vi "Tacking Helper Helper - Starting Angle Test.vi"(6 "Waypoint Array In":T1[](array[typedef]) {"Point Type" items=["Drive", "Round Port", "Round Starboard", "Stay"]}, 9 "Starting Arm Length":dbl, 10 "Tests whether the while\nloop is on its first step":bool, 11 "Step Number\nof While Loop":i32) -> (3 "Boolean out":bool)   [LabVIEW 2011]
uses:
  2x3-RIO-OCU Comm/2x3 Typedefs/ocuWaypoint.ctl
  2x3-RIO-OCU Comm/2x3 Typedefs/waypointTypes.ctl
  2 Typedefs/UTM Location.ctl
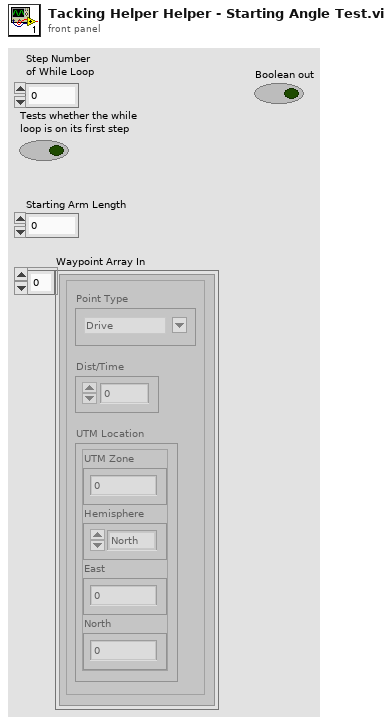
[diagram p1: front panel]
types:
  T1 = typedef "ocuWaypoint.ctl" = cluster{"Point Type":T2, "Dist/Time":dbl, "UTM Location":T3}
  T2 = typedef "waypointTypes.ctl" = u16
  T3 = typedef "UTM Location.ctl" = cluster{"UTM Zone":dbl, "Hemisphere":enum16{"North", "South"}, "East":dbl, "North":dbl}
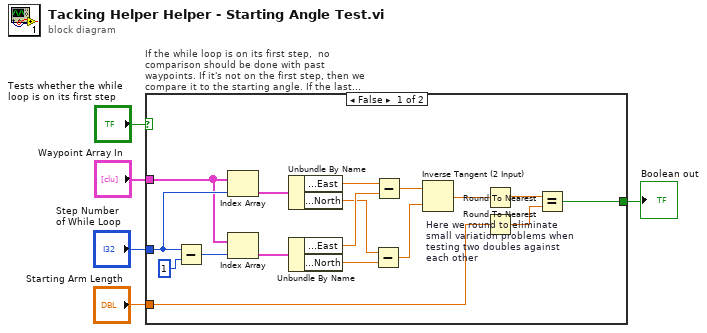
[diagram p0: block diagram]
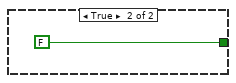
[diagram p2: hidden frame]
diagram:
  n1 = case "If the while loop is on its first step,  no comparison should be done with past waypoints. If it's not on the first step, then we compare it to the starting angle. If the last angle used was\nthe starting angle, true is returned and we use the starting angle again next" shown="False" "Tests whether the while\nloop is on its first step" {
    tunnel: "Waypoint Array In" -> [w10 _]
    tunnel: "Step Number\nof While Loop" -> [w12 _]
    tunnel: "Starting Arm Length" -> [w9 _]
    tunnel: [w11 FALSE] -> w5
    frame False {
      n2 = Subtract(x=w12, y=1 ("x")) -> (x-y=w22:i32)
      n3 = Index Array(array=w10, index=w12) -> (element=w21:T1)
      n4 = Index Array(array=w10, index=w22) -> (element=w20:T1)
      n5 = Unbundle By Name(w21) -> ("UTM Location.East"=w18:dbl, "UTM Location.North"=w17:dbl)
      n6 = Unbundle By Name(w20) -> ("UTM Location.East"=w19:dbl, "UTM Location.North"=w16:dbl)
      n7 = Subtract(x=w17, y=w16) -> (x-y=w15:dbl)
      n8 = Subtract(x=w18, y=w19) -> (x-y=w14:dbl)
      n9 = Inverse Tangent (2 Input)(1:w15, 2:w14) -> (0:w6:dbl)
      n10 = Round To Nearest "Here we round to eliminate\nsmall variation problems when\ntesting two doubles against\neach other"(number=w6) -> (nearest integer value=w7:dbl)
      n11 = Round To Nearest(number=w9) -> (nearest integer value=w8:dbl)
      n12 = Equal?(x=w7, y=w8) -> (x = y?=w11:bool)
    }
    frame True {
    }
  }
  "Boolean out" <- w5
